vi "Add Item.vi"(8 "错误输入":errorcluster, 9 "Mode":enum16{"End", "Begin"}(ring), 10 "Item":string[](array[string]), 11 "Mlistbox Ref":refnum<vi>) -> (0 "错误输出":errorcluster, 3 "Mlistbox Ref Dup":refnum<vi>)   [LabVIEW 2012, in "Mlistbox Tools.lvlib"]
uses:
  Mlistbox Tools.lvlib
  ListBox/Custom Type/Read and Write Mode.ctl
  Property/Set and Get ItemNames.vi
  ListBox/Listbox Tool.lvlib
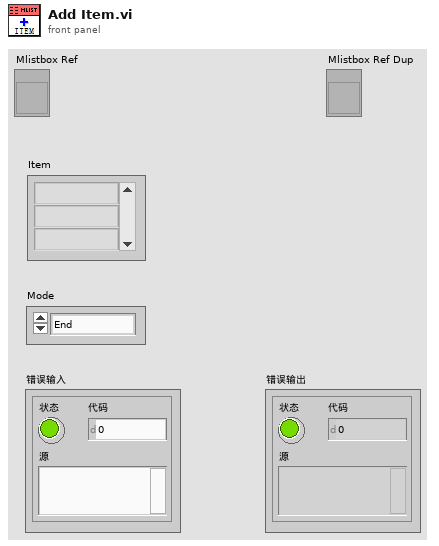
[diagram p1: front panel]
types:
  T1 = typedef "Listbox Tool.lvlib/Read and Write Mode.ctl" = enum16{"Read", "Write"}
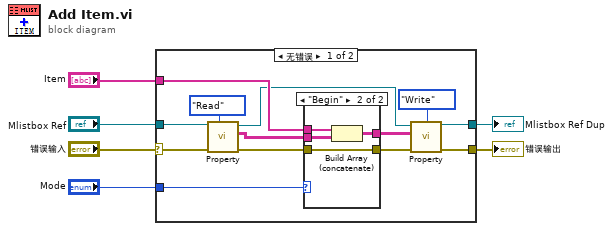
[diagram p0: block diagram]
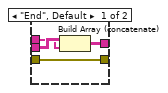
[diagram p2: hidden frame]
diagram:
  n1 = case shown="无错误" "错误输入" {
    selector: "错误输入" -> [w12 w29]
    tunnel: [w10 w29] -> w5
    tunnel: "Mlistbox Ref" -> [w19 w28]
    tunnel: "Mode" -> [w17 _]
    tunnel: "Item" -> [w15 _]
    tunnel: [w11 w28] -> w1
    frame No Error {
      n2 = call-poly "Property.vi"("Mode"=Read_and_Write_Mode."Read", "错误输入"=w12, "Mlistbox Ref"=w19) -> ("错误输出"=w9:errorcluster, "ItemNames Out"=w16:string[][], "Mlistbox Ref Dup"=w7:refnum<vi>)  [unwired: 6 in]
      n3 = case shown="\"Begin\"" w17 {
        tunnel: w16 -> [w23 w26]
        tunnel: w15 -> [w22 w27]
        tunnel: [w21 w25] -> w13
        tunnel: w9 -> [w20 w24]
        tunnel: [w20 w24] -> w8
        frame "End", Default {
          n4 = Build Array (concatenate)(w23, w22) -> (w21:string[][])
        }
        frame "Begin" {
          n5 = Build Array (concatenate)(w27, w26) -> (w25:string[][])
        }
      }
      n6 = call-poly "Property.vi"("Mode"=Read_and_Write_Mode."Write", "错误输入"=w8, "ItemNames In"=w13, "Mlistbox Ref"=w7) -> ("错误输出"=w10:errorcluster, "Mlistbox Ref Dup"=w11:refnum<vi>)  [unwired: 5 in, 1 out]
    }
    frame Error {
    }
  }
  "Mlistbox Ref Dup" <- w1
  "错误输出" <- w5
